vi "S30c_dll build error cluster.vi"(4 "error in":errorcluster, 5 "error Text":string, 6 "error code":i16, 7 "Dev Addr":u8) -> (0 "error out":errorcluster)   [LabVIEW 2014, in "K_S30c_dll.lvlib"]
uses:
  K_S30c_dll.lvlib
panel:
  # "Build error cluster for error-codes from the s30c.dll\nKeller AG für Druckmesstechnik 2008 bv\n29.5.08 b.v."
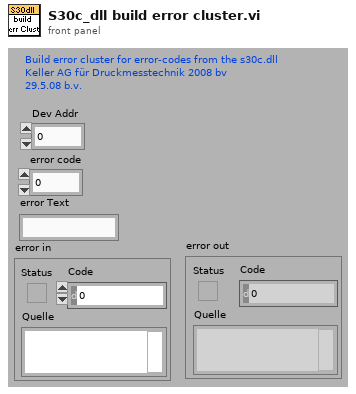
[diagram p1: front panel]
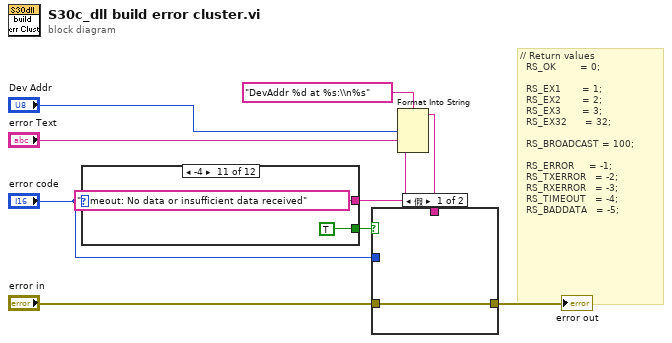
[diagram p0: block diagram]
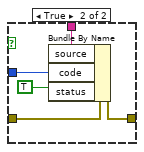
[diagram p2: hidden frame]
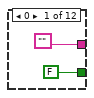
[diagram p3: hidden frame]
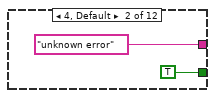
[diagram p4: hidden frame]
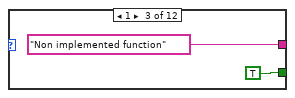
[diagram p5: hidden frame]
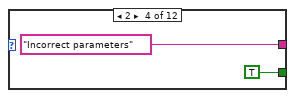
[diagram p6: hidden frame]
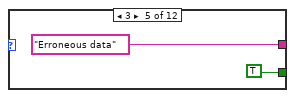
[diagram p7: hidden frame]
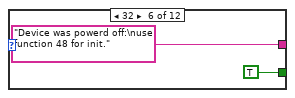
[diagram p8: hidden frame]
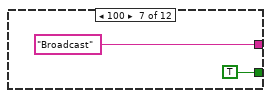
[diagram p9: hidden frame]
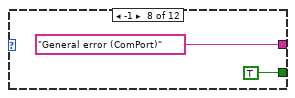
[diagram p10: hidden frame]
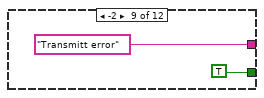
[diagram p11: hidden frame]
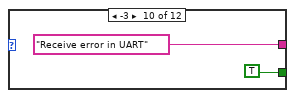
[diagram p12: hidden frame]
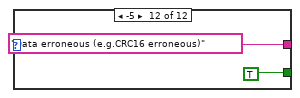
[diagram p13: hidden frame]
diagram:
  # "// Return values\n  RS_OK        = 0;\n\n  RS_EX1       = 1;\n  RS_EX2       = 2;\n  RS_EX3       = 3;\n  RS_EX32      = 32;\n\n  RS_BROADCAST = 100;\n\n  RS_ERROR     = -1;\n  RS_TXERROR   = -2;\n  RS_RXERROR   = -3;\n  RS_TIMEOUT   = -4;\n  RS_BADDATA   = -5;"
  n1 = case shown="-4" "error code" {
    tunnel: ["" "unknown error" "Non implemented function" "Incorrect parameters" "Erroneous data" "Device was powerd off:\nuse function 48 for init." "Broadcast" "General error (ComPort)" "Transmitt error" "Receive error in UART" "Timeout: No data or insufficient data received" "Data erroneous (e.g.CRC16 erroneous)"] -> w3
    tunnel: [FALSE ("status") TRUE TRUE ("status") TRUE ("status") TRUE ("status") TRUE ("status") TRUE ("status") TRUE ("status") TRUE ("status") TRUE ("status") TRUE ("status") TRUE ("status")] -> w1
    frame 0 {
    }
    frame 4, Default {
    }
    frame 1 {
    }
    frame 2 {
    }
    frame 3 {
    }
    frame 32 {
    }
    frame 100 {
    }
    frame -1 {
    }
    frame -2 {
    }
    frame -3 {
    }
    frame -4 {
    }
    frame -5 {
    }
  }
  n2 = Format Into String(format string="DevAddr %d at %s:\\n%s" ("Format-String"), "Dev Addr", "error Text", w3) -> (resulting string=w2:string)  [unwired: 2 in, 1 out]
  n3 = case shown="假" w1 {
    tunnel: "error in" -> [w34 w39]
    tunnel: "error code" -> [_ w38]
    tunnel: w2 -> [_ w37]
    tunnel: [w34 w36] -> w6
    frame False {
    }
    frame True {
      n4 = Bundle By Name(cluster=w39, "source"=w37, "code"=w38, "status"=TRUE) -> (w36:errorcluster)
    }
  }
  "error out" <- w6
